vi "DAQ_Analog_Input.vi"(8 "error in":errorcluster) -> (0 "error out":errorcluster)   [LabVIEW 2025]
panel:
  in  "# or repetitions":u32=2 min=2 step=1
  out "Slide":u32(slide) scale=0.0..100.0
  out "Time per frame":u32
  in  "Scanning parameters":cluster{"Nb pts X":u32, "Nb pts Y":u32}={"Nb pts X"=100, "Nb pts Y"=100}
  in  "AI Range (V)":cluster{"AImin":dbl, "AImax":dbl}={"AImin"=-10.0, "AImax"=10.0}
  out "Image AI0":dbl[][](graph)
  in  "Analog Input Channel(s)":tag="USB-6363/ai0"
  in  "Quit":bool
  in  "Pixel dwelltime (s)":dbl=1e-05 format="%#_6p"
  in  "Trig terminal":tag="/USB-6363/PFI12"
  # "Il faut brancher sur une entrée de compteur un signal TTL"
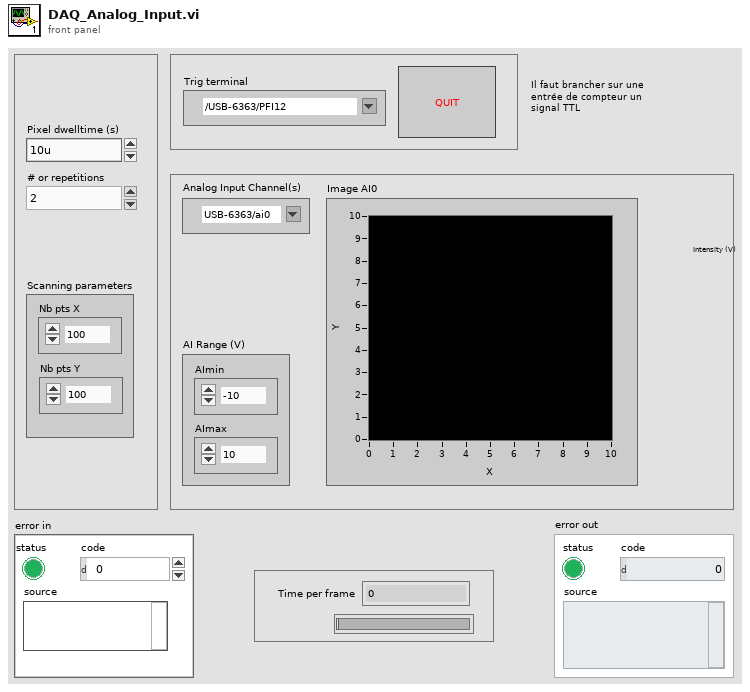
[diagram p1: front panel]
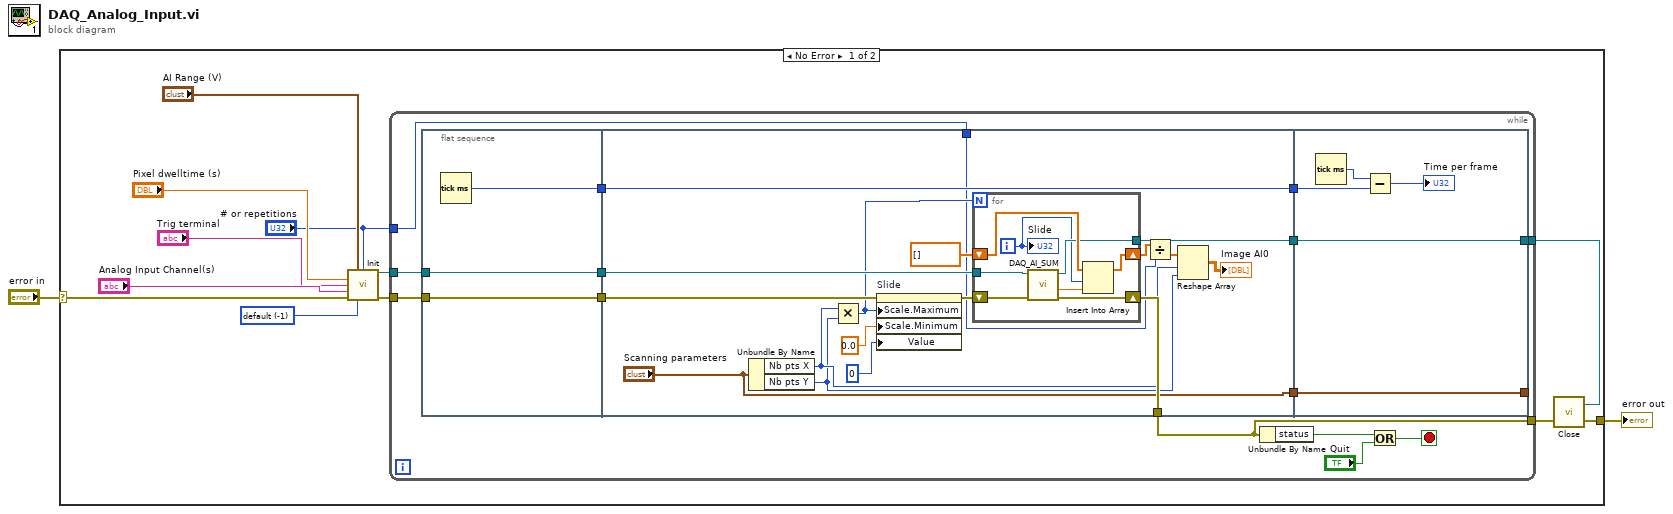
[diagram p0: block diagram]
diagram:
  n1 = case shown="No Error" "error in" {
    selector: "error in" -> [w5 w62]
    tunnel: [w6 w62] -> w2
    frame No Error {
      w8 = -1 items=["default"=-1, "RSE"=10083, "NRSE"=10078, "Differential"=10106, "Pseudodifferential"=12529] ("input terminal configuration")
      n2 = call "Init.vi"("AI Range (V)"="AI Range (V)", "Repetitions"="# or repetitions", "Pixel Dwell time (s)"="Pixel dwelltime (s)", "Trigger terminal"="Trig terminal", "AI Channels"="Analog Input Channel(s)", "error in"=w5, "input terminal configuration"=w8) -> ("AI Task out"=w9:refnum<k21>, "error out"=w11:errorcluster)  [unwired: 7 in]
      n3 = while {
        tunnel: w9 -> [w22]
        tunnel: w11 -> [w28]
        tunnel: [w27] -> w7
        tunnel: [w23] -> w14
        tunnel: "# or repetitions" -> [w15]
        stop <- w24 stop-if-true
        n4 = flat-sequence {
          tunnel: w22 -> [w30]
          tunnel: w28 -> [w31]
          tunnel: [w31] -> w21
          tunnel: [w30] -> w20
          tunnel: [w29] -> w17
          tunnel: [w47] -> w23
          tunnel: w21 -> [w41]
          tunnel: w20 -> [w46]
          tunnel: [w48] -> w19
          tunnel: ["Scanning parameters"] -> w18
          tunnel: w17 -> [w43]
          tunnel: [w43] -> w16
          tunnel: w15 -> [w32]
          tunnel: [w60] -> _
          tunnel: [w61] -> w27
          tunnel: w19 -> [w61]
          tunnel: w18 -> [w60]
          tunnel: w16 -> [w58]
          frame #0 {
            n5 = Tick Count (ms)() -> (millisecond timer value=w29:u32)
          }
          frame #1 {
            n6 = Unbundle By Name("Scanning parameters") -> ("Nb pts X"=w39:u32, "Nb pts Y"=w38:u32)
            n7 = Multiply(x=w39, y=w38) -> (x*y=w35:u32)
            n8 = property on="Slide" class="Slide (strict)"(error in=w41, "Scale.Maximum"=w35, "Scale.Minimum"=0.0 ("Scale.Range:Minimum"), "Value"=u32 0 ("Slide")) -> (error out=w40:errorcluster)  [unwired: 1 in, 1 out]
            n9 = for {
              N: w35 -> [_]
              shift-right: [w55] -> w47
              shift-left: w40 -> [w56]
              tunnel: w46 -> [w51]
              tunnel: [w50] -> w48
              shift-right: [w52] -> w33
              shift-left: dbl[] [] -> [w54]
              i -> [w49]
              n10 = call "DAQ_AI_SUM.vi"("error in"=w56, "AI Task in"=w51) -> ("error out"=w55:errorcluster, "data"=w53:dbl, "AI Task out"=w50:refnum<k21>)  [unwired: 4 in]
              n11 = Insert Into Array(array=w54, index=w49, new element=w53) -> (w52:dbl[])
              "Slide" <- w49
            }
            n12 = Divide(x=w33, y=w32) -> (x/y=w34:dbl[])
            n13 = Reshape Array(w34, w39, w38) -> (→"Image AI0":dbl[][])
          }
          frame #2 {
            n14 = Tick Count (ms)() -> (millisecond timer value=w59:u32)
            n15 = Subtract(x=w59, y=w58) -> (x-y=→"Time per frame":u32)
          }
        }
        n16 = Unbundle By Name(w23) -> ("status"=w26:bool)
        n17 = Or(x=w26, y="Quit") -> (x .or. y?=w24:bool)
      }
      n18 = call "Close.vi"("error in"=w14, "AI Task in"=w7) -> ("error out"=w6:errorcluster)  [unwired: 1 in]
    }
    frame Error {
    }
  }
  "error out" <- w2
